vi "CBL Config.vi"(7 "pCmdList":T1, 8 "error in (no error)":errorcluster, 9 "pInitConfig":T2, 10 "CANIndex":i32, 11 "DevIndex":i32) -> (0 "error out":errorcluster, 3 "function return":i32)   [LabVIEW 2012, in "CANBootloader.lvlib"]
doc: "int WINAPI CBL_Config(int DevIndex,int CANIndex,PVCI_INIT_CONFIG_EX pInitConfig,PCBL_CMD_LIST pCmdList);"
uses:
  CANBootloader.lvlib
  Ginkgo_Driver.dll
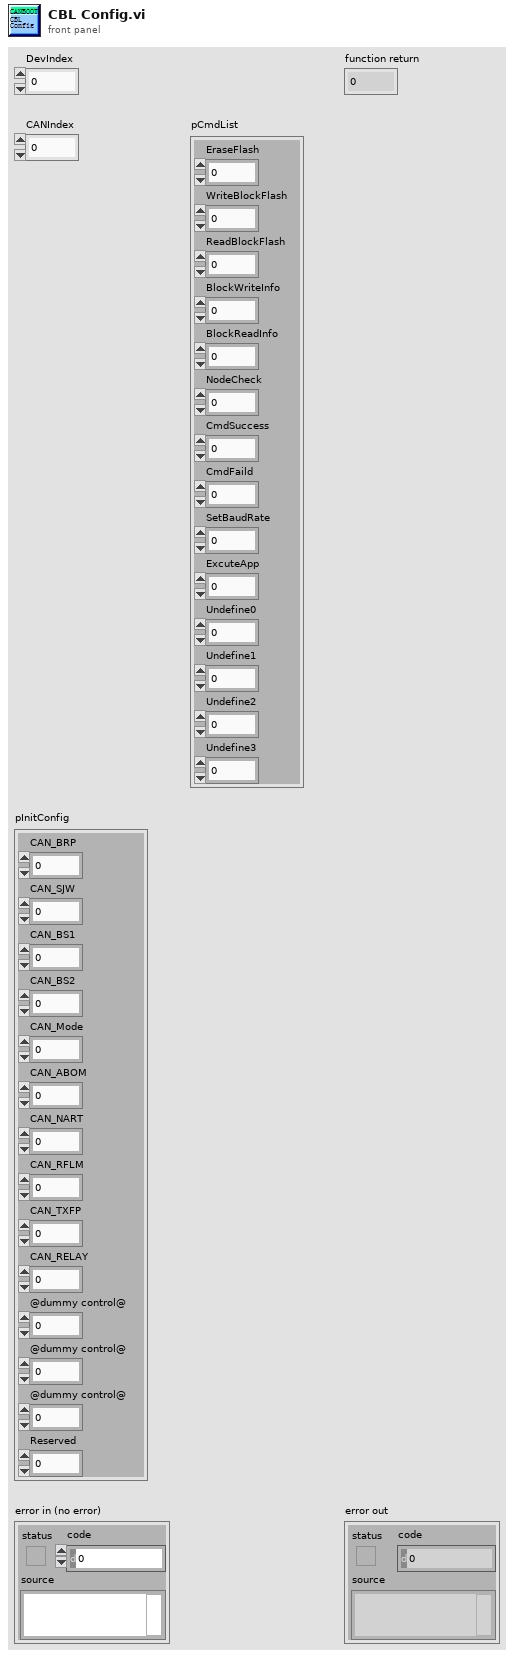
[diagram p1: front panel]
types:
  T1 = cluster{"EraseFlash":u8, "WriteBlockFlash":u8, "ReadBlockFlash":u8, "BlockWriteInfo":u8, "BlockReadInfo":u8, "NodeCheck":u8, "CmdSuccess":u8, "CmdFaild":u8, "SetBaudRate":u8, "ExcuteApp":u8, "Undefine0":u8, "Undefine1":u8, "Undefine2":u8, "Undefine3":u8}
  T2 = cluster{"CAN_BRP":u32, "CAN_SJW":u8, "CAN_BS1":u8, "CAN_BS2":u8, "CAN_Mode":u8, "CAN_ABOM":u8, "CAN_NART":u8, "CAN_RFLM":u8, "CAN_TXFP":u8, "CAN_RELAY":u8, "@dummy control@":i8, "@dummy control@":i8, "@dummy control@":i8, "Reserved":u32}
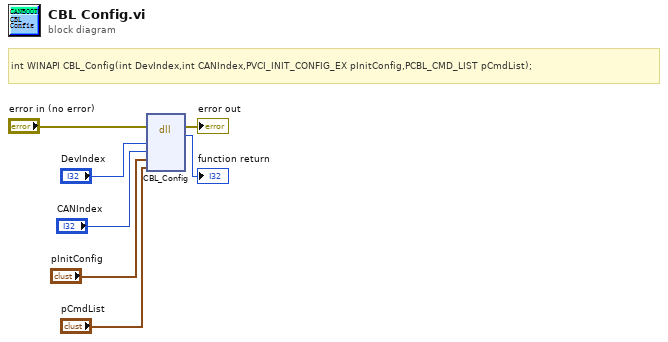
[diagram p0: block diagram]
diagram:
  # "int WINAPI CBL_Config(int DevIndex,int CANIndex,PVCI_INIT_CONFIG_EX pInitConfig,PCBL_CMD_LIST pCmdList);"
  n1 = dll-call lib="E:/Project/vt_ginkgo/truck/Ginkgo Driver/vs2010/Ginkgo_USB-I2C_API_v2.0.3.0/lib/labview_64bit/CANBootloader/Ginkgo_Driver.*" fn="CBL_Config"(error in="error in (no error)", "DevIndex"="DevIndex", "CANIndex"="CANIndex", "pInitConfig"="pInitConfig", "pCmdList"="pCmdList") -> (error out=→"error out":errorcluster, →"function return":i32)  [unwired: 6 in, 1 out]
